vi "Stop Core.vi"(10 "final error code":i32, 11 "Cap Bank Server in":refnum<class "Cap Bank Server.lvclass">) -> (3 "Cap Bank Server out":refnum<class "Cap Bank Server.lvclass">)   [LabVIEW 2012, in "Cap Bank Server.lvclass"]
uses:
  Cap Bank Server.lvclass
  Mag Lab Measure Controller.lvclass
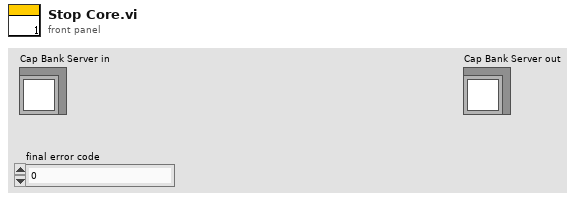
[diagram p1: front panel]
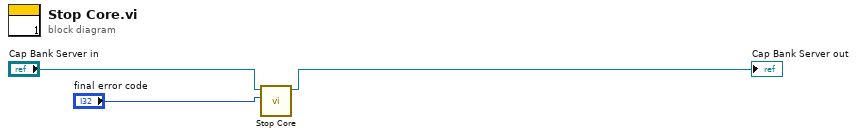
[diagram p0: block diagram]
diagram:
  n1 = call-parent "Stop Core.vi"("final error code"="final error code", "Mag Lab Measure Controller in"="Cap Bank Server in") -> ("Mag Lab Measure Controller out"=→"Cap Bank Server out":refnum<class "Cap Bank Server.lvclass">)  [unwired: 9 in]
